vi "Auto Recock Winch.vi"(11 "Run?":bool) -> (3 "Done":bool)   [LabVIEW 2013]
uses:
  <vilib>/addons/control/pid/pid.llb/PID (DBL).vi
  <vilib>/addons/control/pid/NI_PID_pid.lvlib
panel:
  in  "PID gains":T1={"proportional gain (Kc)"=2.75, "integral time (Ti, min)"=0.0, "derivative time (Td, min)"=0.0} {"derivative time (Td, min)" format="%.3f"; "integral time (Ti, min)" format="%.3f"; "proportional gain (Kc)" format="%.3f"}
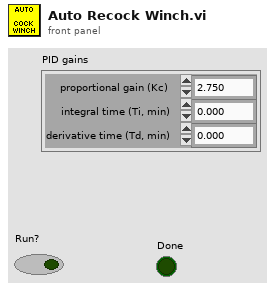
[diagram p1: front panel]
types:
  T1 = cluster{"proportional gain (Kc)":dbl, "integral time (Ti, min)":dbl, "derivative time (Td, min)":dbl}
  T2 = typedef "WPI_DigitalInputDevRef.ctl" = cluster{"DevStatus":errorcluster, "DIO Channel":T3, "Digital Module":T4}
  T3 = typedef "FPGA_DIOChannel.ctl" = enum8{"DIO 1", "DIO 2", "DIO 3", "DIO 4", "DIO 5", "DIO 6", "DIO 7", "DIO 8", "DIO 9", "DIO 10", "DIO 11", "DIO 12", "DIO 13", "DIO 14", "Invalid"}
  T4 = typedef "FPGA_TypedefDigitalModule.ctl" = enum16{"Digital Module 1", "Digital Module 2"}
  T5 = typedef "WPI_MotorControlDeviceRef.ctl" = cluster{"DeviceStatus":errorcluster, "Type":enum16{"PWM", "CAN"}, "PWM":cluster{"Digital Module":T4, "PWM Channel":T6, "DeadBand":T7}, "CAN":cluster{"Device Number":u8, "Control Mode":T8, "Semaphore":T9, "Max Vout":dbl}, "Invert":bool, "TransformRef":T10, "InvTransformRef":T10}
  T6 = typedef "FPGA_DIOPWMChannel.ctl" = enum8{"PWM 1", "PWM 2", "PWM 3", "PWM 4", "PWM 5", "PWM 6", "PWM 7", "PWM 8", "PWM 9", "PWM 10", "Invalid"}
  T7 = typedef "WPI_PWMDeadband.ctl" = cluster{"Name":string, "maxPositivePwm":i32, "minPositivePwm":i32, "centerPwm":i32, "maxNegativePwm":i32, "minNegativePwm":i32, "angularRange":u16}
  T8 = typedef "WPI_CANJaguar_ControlMode.ctl" = enum8{"Percent VBus", "Current", "Speed", "Position", "Voltage"}
  T9 = typedef "Semaphore RefNum" = refnum<k1>
  T10 = typedef "WPI_PWMTransform_ConPane.ctl" = refnum<vi>
  T11 = typedef "WPI_AnalogChannelDevRef.ctl" = cluster{"DevStatus":errorcluster, "Analog Module":T12, "Analog Channel":T13}
  T12 = typedef "FPGA_TypedefAnalogModule.ctl" = enum16{"Analog Module 1", "Analog Module 2"}
  T13 = typedef "FPGA_AIChannel.ctl" = enum8{"AI 1", "AI 2", "AI 3", "AI 4", "AI 5", "AI 6", "AI 7", "AI 8", "Invalid"}
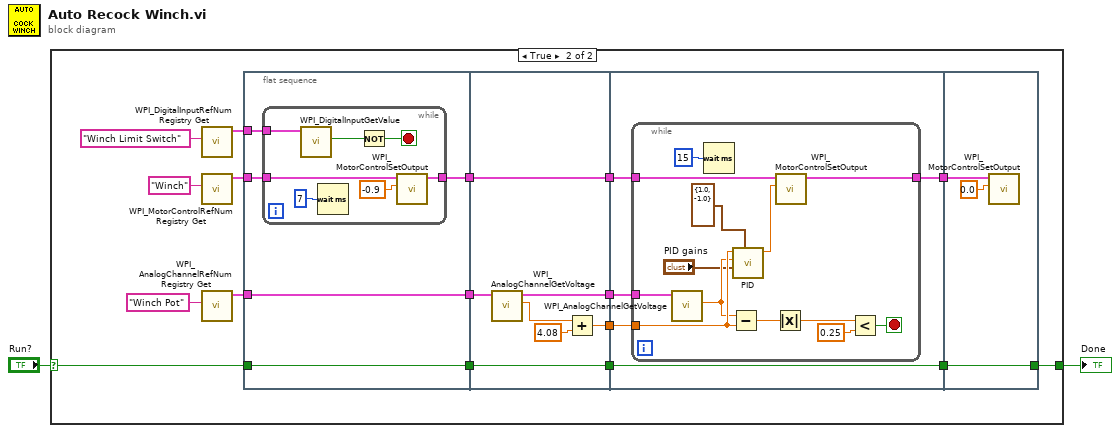
[diagram p0: block diagram]
diagram:
  n1 = case shown="True" "Run?" {
    selector: "Run?" -> [w3 w8]
    tunnel: [w3 w4] -> w1
    frame False {
    }
    frame True {
      n2 = call <vilib>:"WPI_DigitalInputRefNum Registry Get.vi"("refnum name"="Winch Limit Switch") -> ("DigitalInputDevRef"=w12:T2)  [unwired: 9 in, 1 out]
      n3 = call <vilib>:"WPI_MotorControlRefNum Registry Get.vi"("refnum name"="Winch") -> ("MotorControlDevRef"=w13:T5)  [unwired: 9 in, 1 out]
      n4 = call <vilib>:"WPI_AnalogChannelRefNum Registry Get.vi"("refnum name"="Winch Pot") -> ("AIDeviceRef"=w14:T11)  [unwired: 9 in, 1 out]
      n5 = flat-sequence {
        tunnel: w12 -> [w25]
        tunnel: w13 -> [w24]
        tunnel: [w23] -> w20
        tunnel: [w22] -> w19
        tunnel: w14 -> [w22]
        tunnel: w8 -> [w21]
        tunnel: [w21] -> w7
        tunnel: w20 -> [w39]
        tunnel: [w39] -> w18
        tunnel: [w38] -> w17
        tunnel: w19 -> [w37]
        tunnel: [w35] -> w16
        tunnel: w7 -> [w33]
        tunnel: [w33] -> w6
        tunnel: w18 -> [w44]
        tunnel: w17 -> [w42]
        tunnel: [w41] -> w15
        tunnel: w16 -> [w43]
        tunnel: w6 -> [w40]
        tunnel: [w40] -> w5
        tunnel: w15 -> [w60]
        tunnel: w5 -> [w58]
        tunnel: [w58] -> w4
        frame #0 {
          n6 = while {
            tunnel: w25 -> [w32]
            tunnel: w24 -> [w29]
            tunnel: [w28] -> w23
            stop <- w27 stop-if-true
            n7 = call <vilib>:"WPI_DigitalInputGetValue.vi"("DigitalInputDevRef"=w32) -> ("Value"=w31:bool)  [unwired: 8 in, 2 out]
            n8 = Wait (ms)(milliseconds to wait=u32 7) -> ()  [unwired: 1 out]
            n9 = Not(x=w31) -> (.not. x?=w27:bool)
            n10 = call <vilib>:"WPI_MotorControlSetOutput.vi"("Output"=-0.9, "MotorControlDevRef"=w29) -> ("MotorControlDevRef"=w28:T5)  [unwired: 7 in, 2 out]
          }
        }
        frame #1 {
          n11 = call <vilib>:"WPI_AnalogChannelGetVoltage.vi"("AIDeviceRef"=w37) -> ("Voltage"=w36:dbl, "AIDeviceRef"=w38:T11)  [unwired: 8 in, 1 out]
          n12 = Add(x=w36, y=4.08) -> (x+y=w35:dbl)
        }
        frame #2 {
          n13 = while {
            tunnel: w44 -> [w57]
            tunnel: w43 -> [w50]
            tunnel: w42 -> [w52]
            tunnel: [w48] -> w41
            stop <- w54 stop-if-true
            n14 = call <vilib>:"WPI_AnalogChannelGetVoltage.vi"("AIDeviceRef"=w52) -> ("Voltage"=w49:dbl)  [unwired: 8 in, 2 out]
            n15 = Wait (ms)(milliseconds to wait=u32 15) -> ()  [unwired: 1 out]
            n16 = Subtract(x=w49, y=w50) -> (x-y=w56:dbl)
            n17 = call-poly <vilib>:"PID.vi"("output range"=cluster{"output high":dbl, "output low":dbl} {"output high"=1.0, "output low"=-1.0}, "PID gains"="PID gains", "process variable"=w49, "setpoint"=w50) -> ("output"=w46:dbl)  [unwired: 6 in, 1 out]
            n18 = Absolute Value(x=w56) -> (abs(x)=w55:dbl)
            n19 = call <vilib>:"WPI_MotorControlSetOutput.vi"("Output"=w46, "MotorControlDevRef"=w57) -> ("MotorControlDevRef"=w48:T5)  [unwired: 7 in, 2 out]
            n20 = Less?(x=w55, y=0.25) -> (x < y?=w54:bool)
          }
        }
        frame #3 {
          n21 = call <vilib>:"WPI_MotorControlSetOutput.vi"("Output"=0.0, "MotorControlDevRef"=w60) -> ()  [unwired: 7 in, 3 out]
        }
      }
    }
  }
  "Done" <- w1
